vi "Puzzle 2-2.vi"() -> ()   [LabVIEW 2022 SP3]
panel:
  out "sum":i32
  out "Array":string[](array[string])
  in  "delimited string":string
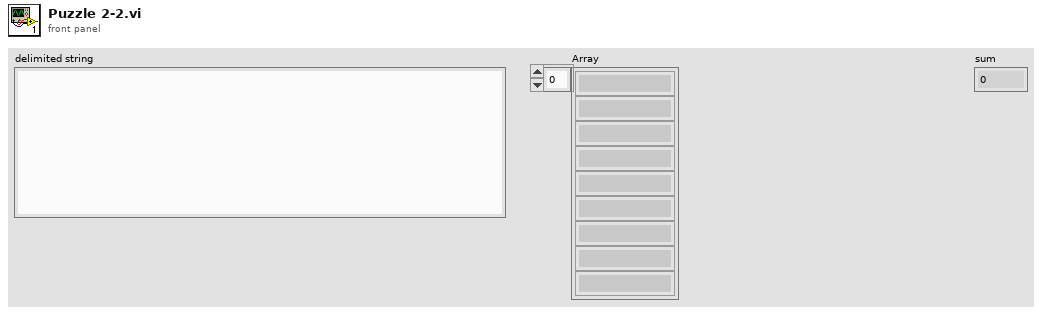
[diagram p1: front panel]
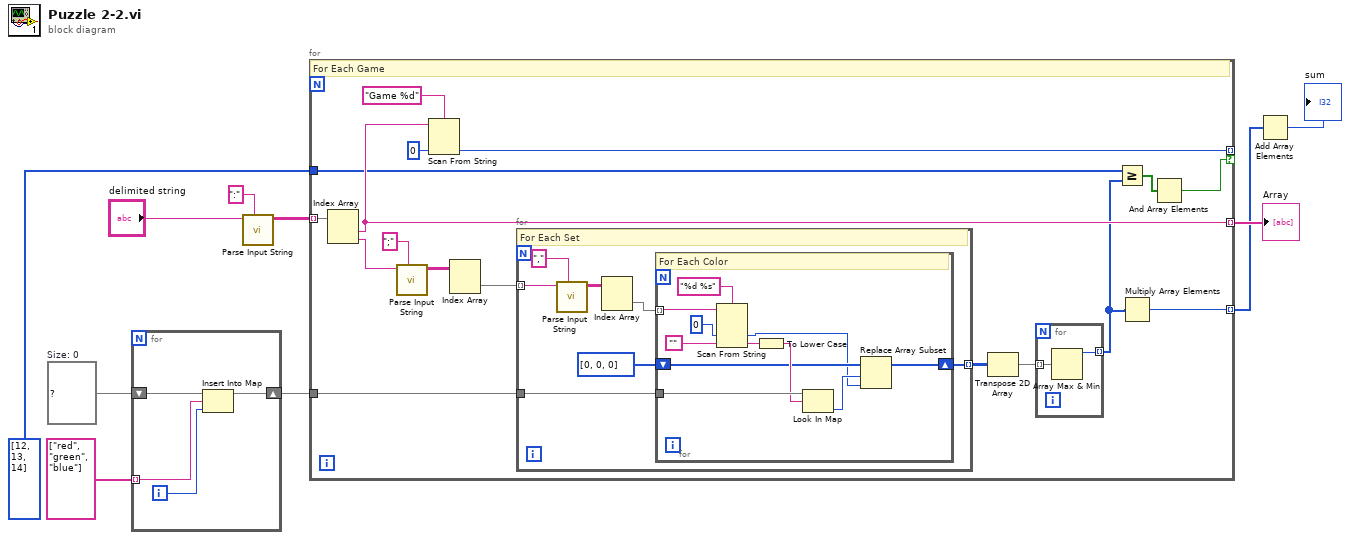
[diagram p0: block diagram]
diagram:
  w6 = map{string, i32} {}  # Size: 0
  n1 = for {
    shift-right: [w12] -> w4
    shift-left: w6 -> [w14]
    tunnel: string[] ["red", "green", "blue"] -> [w13] mode=indexing
    i -> [w11]
    n2 = Insert Into Map(map in=w14, key=w13, value=w11) -> (map out=w12:map{string, i32})  [unwired: 2 out]
  }
  n3 = call "Parse Input String.vi"("delimiter (Tab)"=":", "delimited string"="delimited string") -> ("parsed string"=w8:string[][])  [unwired: 9 in]
  n4 = for {
    tunnel: w8 -> [w30] mode=indexing
    tunnel: [w26] -> w7 mode=indexing
    tunnel: [w23] -> _ mode=indexing if=w17
    tunnel: w4 -> [w22]
    tunnel: i32[] [12, 13, 14] -> [w19]
    tunnel: [w15] -> w1 mode=indexing
    # "For Each Game"
    n5 = Index Array(array=w30) -> (element #1=w26:string, element #2=w29:string)  [unwired: 2 in]
    n6 = call "Parse Input String.vi"("delimiter (Tab)"=";", "delimited string"=w29) -> ("parsed string"=w28:string[][])  [unwired: 9 in]
    n7 = Scan From String(format string="Game %d", input string=w26, default 1=0 ("default value 1")) -> (output 1=w23:i32)  [unwired: 2 in, 3 out]
    n8 = Index Array(array=w28) -> (element=w27:string[])  [unwired: 2 in]
    n9 = for {
      tunnel: w27 -> [w39] mode=indexing
      tunnel: w22 -> [w35]
      tunnel: [w34] -> w21 mode=indexing
      # "For Each Set"
      n10 = call "Parse Input String.vi"("delimiter (Tab)"=",", "delimited string"=w39) -> ("parsed string"=w38:string[][])  [unwired: 9 in]
      n11 = Index Array(array=w38) -> (element=w37:string[])  [unwired: 2 in]
      n12 = for {
        tunnel: w37 -> [w50] mode=indexing
        shift-right: [w41] -> w34
        shift-left: i32[] [0, 0, 0] -> [w44]
        tunnel: w35 -> [w46]
        # "For Each Color"
        n13 = Scan From String(format string="%d %s", input string=w50, default 1=0 ("default value 1"), default 2="" ("default value 2")) -> (output 1=w42:i32, output 2=w47:string)  [unwired: 2 in, 3 out]
        n14 = To Lower Case(string=w47) -> (all lower case string=w45:string)
        n15 = Look In Map(map=w46, key=w45) -> (value=w43:i32)  [unwired: 1 in, 1 out]
        n16 = Replace Array Subset(array=w44, new element=w42, index=w43) -> (w41:i32[])
      }
    }
    n17 = Transpose 2D Array(2D array=w21) -> (transposed array=w20:i32[][])
    n18 = for {
      tunnel: w20 -> [w33] mode=indexing
      tunnel: [w32] -> w16 mode=indexing
      n19 = Array Max & Min(array=w33) -> (max value=w32:i32)  [unwired: 3 out]
    }
    n20 = Greater Or Equal?(x=w19, y=w16) -> (x >= y?=w18:bool[])
    n21 = Multiply Array Elements(1:w16) -> (0:w15:i32)
    n22 = And Array Elements(Boolean array=w18) -> (logical AND=w17:bool)
  }
  "Array" <- w7
  n23 = Add Array Elements(numeric array=w1) -> (sum=→"sum":i32)
